vi "gh-cli Release List.vi"(8 "error in (no error)":errorcluster, 10 "Options":string, 11 "Git in":refnum<class "Git.lvclass">) -> (0 "error out":errorcluster, 2 "Release(s)":string, 3 "Git out":refnum<class "Git.lvclass">)   [LabVIEW 2019, in "Git.lvclass"]
doc: "gh release list [<b>Options</b>]: List releases in a repository\n\n<b>Options</b>\n-L, --limit <int>: Maximum number of items to fetch\n-R, --repo <[HOST/]OWNER/REPO>: Select another repository using the [HOST/]OWNER/REPO format \n\nhttps://cli.github.com/manual/"
uses:
  Git.lvclass
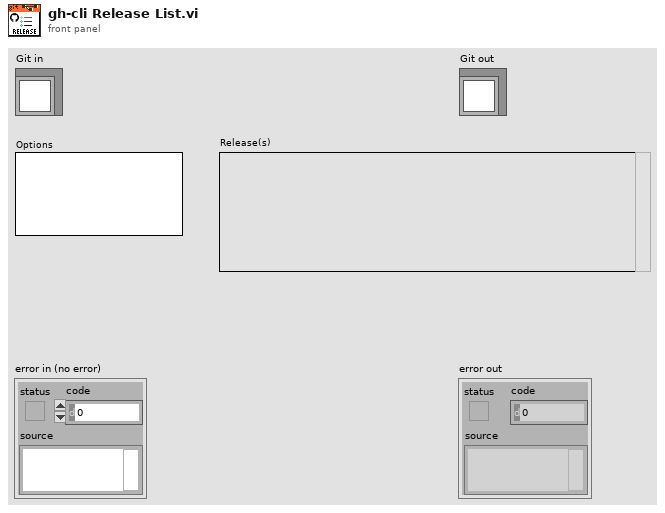
[diagram p1: front panel]
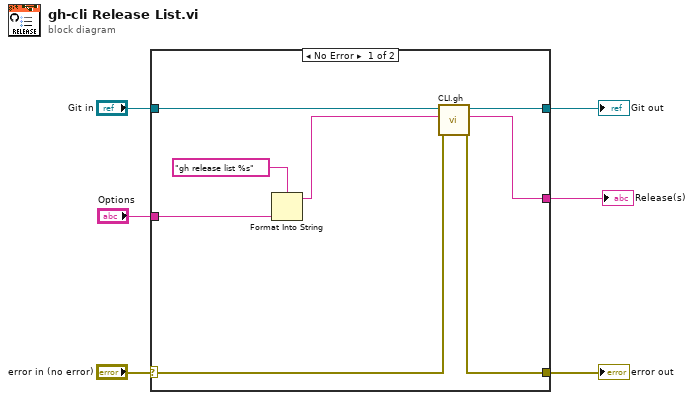
[diagram p0: block diagram]
diagram:
  n1 = case shown="No Error" "error in (no error)" {
    selector: "error in (no error)" -> [w12 w16]
    tunnel: [w11 w16] -> w5
    tunnel: [w13 w15] -> w3
    tunnel: "Git in" -> [w14 w15]
    tunnel: "Options" -> [w9 _]
    tunnel: [w7 _] -> w1
    frame No Error {
      n2 = Format Into String(format string="gh release list %s" ("Command"), w9) -> (resulting string=w8:string)  [unwired: 2 in, 1 out]
      n3 = call "CLI.gh.vi"("error in (no error)"=w12, "Command"=w8, "Git in"=w14) -> ("error out"=w11:errorcluster, "standard output"=w7:string, "Git out"=w13:refnum<class "Git.lvclass">)  [unwired: 4 in, 2 out]
    }
    frame Error {
    }
  }
  "error out" <- w5
  "Git out" <- w3
  "Release(s)" <- w1
